vi "Keep_Last_N_Samples_DBL.vi"(1 "BufferLengthSamples":i32=100, 2 "Input sample":dbl format="%#_13g") -> (0 "Output Array":dbl[](array[numeric]))   [LabVIEW 2018, in "TTL IO.lvlib"]
uses:
  TTL IO.lvlib
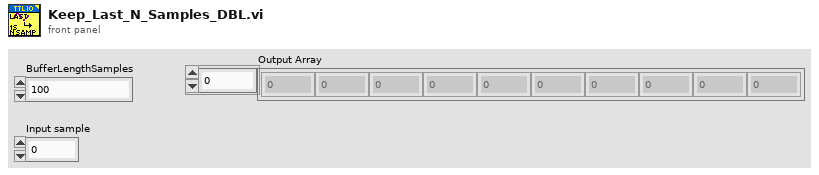
[diagram p1: front panel]
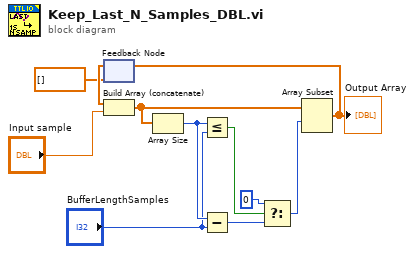
[diagram p0: block diagram]
diagram:
  n1 = feedback #1(dbl[] []) -> (w11:dbl[])
  n2 = Build Array (concatenate)(w11, "Input sample") -> (w10:dbl[])
  n3 = Array Size(array=w10) -> (size(s)=w4:i32)
  n4 = Less Or Equal?(x=w4, y="BufferLengthSamples") -> (x <= y?=w6:bool)
  n5 = Subtract(x=w4, y="BufferLengthSamples") -> (x-y=w2:i32)
  n6 = Select(t=0, s=w6, f=w2) -> (s? t:f=w1:i32)
  n7 = Array Subset(array=w10, index=w1) -> (w9:dbl[])  [unwired: 1 in]
  "Output Array" <- w9
  n8 = feedback-in #1(w9) -> ()
